vi "Measurement Plugin Error Handler.vi"(8 "error in":errorcluster) -> (0 "Errors Out":errorcluster[](array[cluster]), 3 "Status Message (Error)":string)   [LabVIEW 2023]
uses:
  <vilib>/Utility/error.llb/DialogType.ctl
  796815f3-c0a5-4297-8b06-6ee3a6184487.vi
  <vilib>/Utility/error.llb/Trim Whitespace One-Sided.vi
panel:
  out "Error Message Array":string[](array[string])
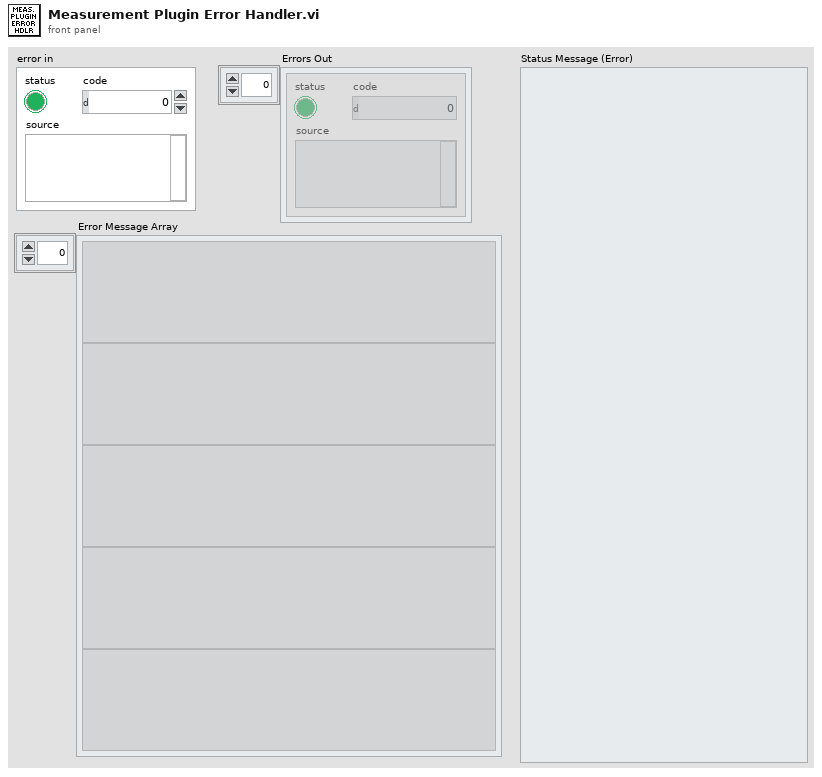
[diagram p1: front panel]
types:
  T1 = typedef "DialogType.ctl" = u16
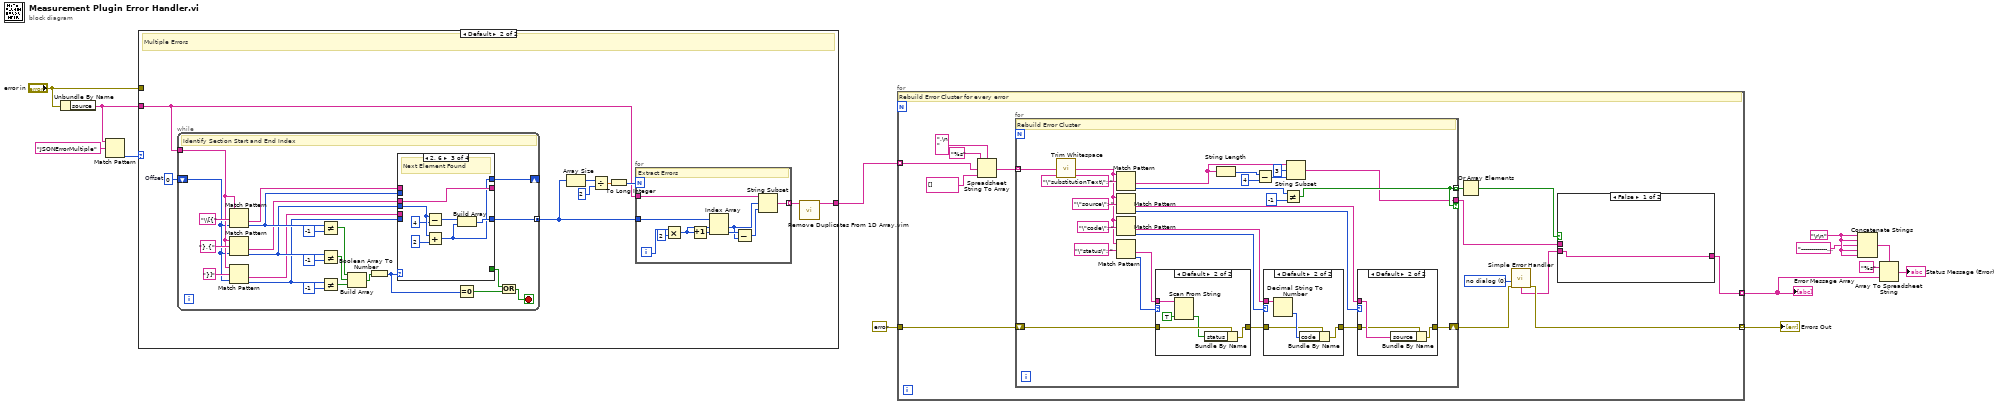
[diagram p0: block diagram]
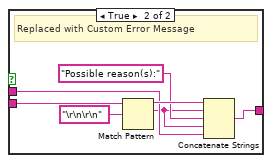
[diagram p2: hidden frame]
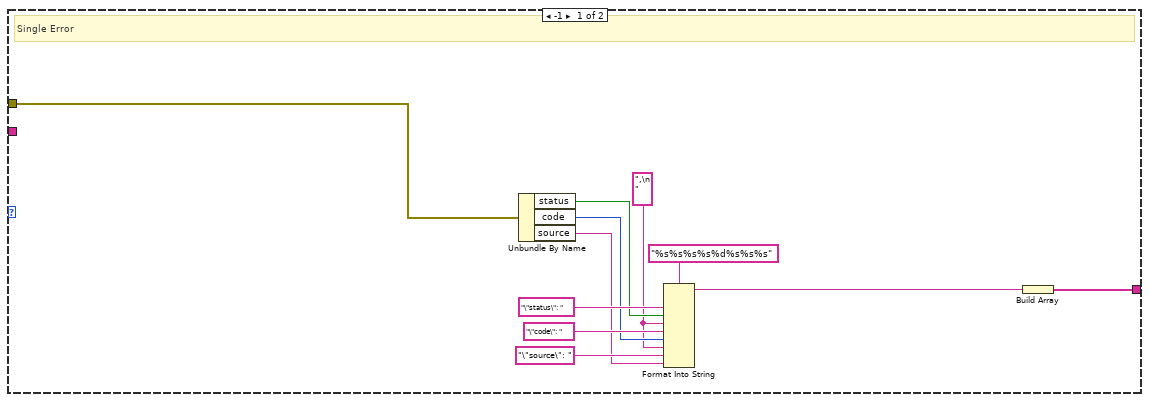
[diagram p6: hidden frame]
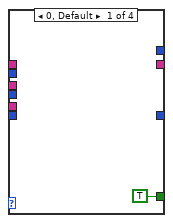
[diagram p7: hidden frame]
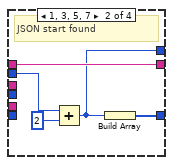
[diagram p8: hidden frame]
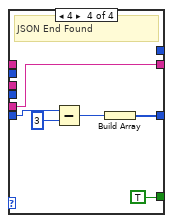
[diagram p9: hidden frame]
diagram:
  w12 = "\r\n"
  n1 = Unbundle By Name("error in") -> ("source"=w5:string)
  n2 = Match Pattern(string=w5, regular expression="JSONErrorMultiple") -> (offset past match=w2:i32)  [unwired: 1 in, 3 out]
  n3 = case shown="Default" w2 {
    tunnel: [w14 w33] -> w6
    tunnel: w5 -> [_ w25]
    tunnel: "error in" -> [w24 _]
    frame -1 {
      w19 = ",\n    " ("delimiter (Tab)")
      # "Single Error"
      n4 = Unbundle By Name(w24) -> ("status"=w22:bool, "code"=w20:i32, "source"=w17:string)
      n5 = Format Into String(format string="%s%s%s%s%d%s%s%s", "\"status\": " ("regular expression"), w22, w19, "\"code\": " ("regular expression"), w20, w19, "\"source\": " ("regular expression"), w17) -> (resulting string=w15:string)  [unwired: 2 in, 1 out]
      n6 = Build Array(w15) -> (w14:string[])
    }
    frame Default {
      w26 = 0  # Offset
      # "Multiple Errors"
      n7 = while {
        tunnel: [w50] -> w30 mode=concatenating
        shift-right: [w48] -> _
        shift-left: w26 -> [w47]
        tunnel: w25 -> [w64]
        stop <- w45 stop-if-true
        # "Identify Section Start and End Index"
        n8 = Match Pattern(string=w64, regular expression="\\[{", offset (0)=w47) -> (after substring=w53:string, offset past match=w56:i32)  [unwired: 2 out]
        n9 = Match Pattern(string=w64, regular expression="},{", offset (0)=w47) -> (after substring=w52:string, offset past match=w55:i32)  [unwired: 2 out]
        n10 = Match Pattern(string=w64, regular expression="}]", offset (0)=w47) -> (after substring=w51:string, offset past match=w54:i32)  [unwired: 2 out]
        n11 = Not Equal?(x=w56, y=-1) -> (x != y?=w59:bool)
        n12 = Not Equal?(x=w55, y=-1) -> (x != y?=w60:bool)
        n13 = Not Equal?(x=w54, y=-1) -> (x != y?=w58:bool)
        n14 = Build Array(w59, w60, w58) -> (w57:bool[])
        n15 = Boolean Array To Number(Boolean array=w57) -> (number=w49:u32)
        n16 = case shown="2, 6" w49 {
          tunnel: w56 -> [_ w72 _ _]
          tunnel: w55 -> [_ _ w77 _]
          tunnel: w54 -> [_ _ _ w85]
          tunnel: w53 -> [_ w73 _ _]
          tunnel: w52 -> [_ _ w80 _]
          tunnel: w51 -> [_ _ _ w86]
          tunnel: [_ w73 w80 w86] -> _
          tunnel: [_ w71 w79 w84] -> w50
          tunnel: [_ w69 w75 _] -> w48
          tunnel: [TRUE _ _ TRUE] -> w44
          frame 0, Default {
          }
          frame 1, 3, 5, 7 {
            # "JSON start found"
            n17 = Add(x=w72, y=2) -> (x+y=w69:i32)
            n18 = Build Array(w69) -> (w71:i32[])
          }
          frame 2, 6 {
            # "Next Element Found"
            n19 = Subtract(x=w77, y=4) -> (x-y=w78:i32)
            n20 = Add(x=w77, y=2) -> (x+y=w75:i32)
            n21 = Build Array(w78, w75) -> (w79:i32[])
          }
          frame 4 {
            # "JSON End Found"
            n22 = Subtract(x=w85, y=3) -> (x-y=w82:i32)
            n23 = Build Array(w82) -> (w84:i32[])
          }
        }
        n24 = Equal To 0?(x=w49) -> (x = 0?=w46:bool)
        n25 = Or(x=w44, y=w46) -> (x .or. y?=w45:bool)
      }
      n26 = Array Size(array=w30) -> (size(s)=w27:i32)
      n27 = Divide(x=w27, y=2) -> (x/y=w28:dbl)
      n28 = To Long Integer(number=w28) -> (32bit integer=w32:i32)
      n29 = for {
        N: w32 -> [_]
        tunnel: [w41] -> w31 mode=indexing
        tunnel: w25 -> [w40]
        tunnel: w30 -> [w34]
        i -> [w43]
        # "Extract Errors"
        n30 = Multiply(x=w43, y=2) -> (x*y=w38:i32)
        n31 = Increment(x=w38) -> (x+1=w42:i32)
        n32 = Index Array(array=w34, index #1=w38, index #2=w42) -> (element #1=w35:i32, element #2=w36:i32)
        n33 = Subtract(x=w36, y=w35) -> (x-y=w39:i32)
        n34 = String Subset(string=w40, offset (0)=w35, length (rest)=w39) -> (substring=w41:string)
      }
      n35 = call "Remove Duplicates From 1D Array.vim"("array"=w31) -> ("array with duplicates removed"=w33:string[])  [unwired: 10 in]
    }
  }
  n36 = for {
    tunnel: w6 -> [w99] mode=indexing
    tunnel: errorcluster {"status"=FALSE, "code"=0, "source"=""} ("error in (no error)") -> [w95]
    tunnel: [w93] -> w7 mode=indexing
    tunnel: [w87] -> w8 mode=indexing
    w91 = T1 0 items=["no dialog", "OK message", "continue or stop message", "OK message + warnings", "continue/stop + warnings"] ("type of dialog (OK msg:1)")
    # "Rebuild Error Cluster for every error"
    n37 = Spreadsheet String To Array(delimiter (Tab)=",\n    ", format string="%s", spreadsheet string=w99, array type (2D Dbl)=string[] []) -> (array=w97:string[])
    n38 = for {
      tunnel: w97 -> [w133] mode=indexing
      shift-right: [w130] -> w94
      shift-left: w95 -> [w127]
      tunnel: [w115] -> w92 mode=indexing
      tunnel: [w109] -> w88 if=w115
      # "Rebuild Error Cluster"
      n39 = call <vilib>:"Trim Whitespace.vi"("string"=w133) -> ("trimmed string"=w118:string)  [unwired: 1 in]
      n40 = Match Pattern(string=w118, regular expression="\"substitutionText\": ") -> (after substring=w114:string, offset past match=w117:i32)  [unwired: 1 in, 2 out]
      n41 = Match Pattern(string=w118, regular expression="\"source\": ") -> (after substring=w131:string, offset past match=w120:i32)  [unwired: 1 in, 2 out]
      n42 = Match Pattern(string=w118, regular expression="\"code\": ") -> (after substring=w123:string, offset past match=w121:i32)  [unwired: 1 in, 2 out]
      n43 = Match Pattern(string=w118, regular expression="\"status\": ") -> (after substring=w124:string, offset past match=w122:i32)  [unwired: 1 in, 2 out]
      n44 = case shown="Default" w122 {
        tunnel: w124 -> [_ w137]
        tunnel: [w134 w139] -> w126
        tunnel: w127 -> [w134 w138]
        frame -1 {
        }
        frame Default {
          n45 = Scan From String(input string=w137, default 1=TRUE) -> (output 1=w136:bool)  [unwired: 3 in, 3 out]
          n46 = Bundle By Name(cluster=w138, "status"=w136) -> (w139:errorcluster)
        }
      }
      n47 = String Length(string=w114) -> (length=w113:i32)
      n48 = Subtract(x=w113, y=4) -> (x-y=w111:i32)
      n49 = case shown="Default" w121 {
        tunnel: w123 -> [_ w144]
        tunnel: [w140 w143] -> w125
        tunnel: w126 -> [w140 w141]
        frame -1 {
        }
        frame Default {
          n50 = Decimal String To Number(string=w144) -> (number=w142:i32)  [unwired: 2 in, 1 out]
          n51 = Bundle By Name(cluster=w141, "code"=w142) -> (w143:errorcluster)
        }
      }
      n52 = Not Equal?(x=w117, y=-1) -> (x != y?=w115:bool)
      n53 = String Subset(string=w114, offset (0)=3, length (rest)=w111) -> (substring=w109:string)
      n54 = case shown="Default" w120 {
        tunnel: w131 -> [_ w147]
        tunnel: [w145 w148] -> w130
        tunnel: w125 -> [w145 w146]
        frame -1 {
        }
        frame Default {
          n55 = Bundle By Name(cluster=w146, "source"=w147) -> (w148:errorcluster)
        }
      }
    }
    n56 = Or Array Elements(Boolean array=w92) -> (logical OR=w89:bool)
    n57 = call <vilib>:"Simple Error Handler.vi"("type of dialog (OK msg:1)"=w91, "error in (no error)"=w94) -> ("error out"=w93:errorcluster, "message"=w90:string)  [unwired: 3 in, 3 out]
    n58 = case shown="False" w89 {
      tunnel: w90 -> [w101 w108]
      tunnel: w88 -> [_ w103]
      tunnel: [w101 w105] -> w87
      frame False {
      }
      frame True {
        # "Replaced with Custom Error Message"
        n59 = Match Pattern(string=w108, regular expression="\r\n\r\n") -> (before substring=w107:string, match substring=w102:string)  [unwired: 1 in, 2 out]
        n60 = Concatenate Strings(w107, w102, "Possible reason(s):" ("regular expression"), w102, w103) -> (w105:string)
      }
    }
  }
  "Error Message Array" <- w8
  "Errors Out" <- w7
  n61 = Concatenate Strings(w12, w12, "-------------------------------------", w12, w12) -> (w13:string)
  n62 = Array To Spreadsheet String(delimiter (Tab)=w13, array=w8, 3:"%s" ("format string")) -> (spreadsheet string=→"Status Message (Error)":string)
